vi "Objects bottom cords.vi"(2 "error in (no error)":errorcluster, 3 "Image":T4) -> (0 "error out":errorcluster, 1 "Objects bottom cords":T3(array[cluster]))   [LabVIEW 2009, in "ImageAnalysis.lvlib"]
doc: "Inputs:\nA binary image where white spotts are objects to detect.\n\nOutput:\nA 1-D array with a cluster element per detected object. Each cluster contains a 1-D array with the detected bottom points of the object."
uses:
  ImageAnalysis.lvlib
  <vilib>/vision/Image Controls.llb/IMAQ Image.ctl
  <vilib>/Analysis/Matrix/Numeric/Conversions/Array To Matrix - RA2.vi
  <vilib>/vision/NI_Vision_Development_Module.lvlib
  <vilib>/Analysis/Matrix/NI_Matrix.lvlib
panel:
  in  "Object":T1
  out "Rectangle":T2 {"Rotation" format="%.2f"; "Left" scale=0.0..1024.0; "Right" scale=0.0..1024.0; "Bottom" scale=1024.0..0.0; "Top" scale=1024.0..0.0}
  in  "Rectangle cluster":T2 {"Rotation" min=-90.0 max=90.0 step=1.0 format="%.2f"; "Left" scale=0.0..1024.0; "Right" scale=0.0..1024.0; "Bottom" scale=1024.0..0.0; "Top" scale=1024.0..0.0}
  # "Excecution time for this node is approx: 350 ms"
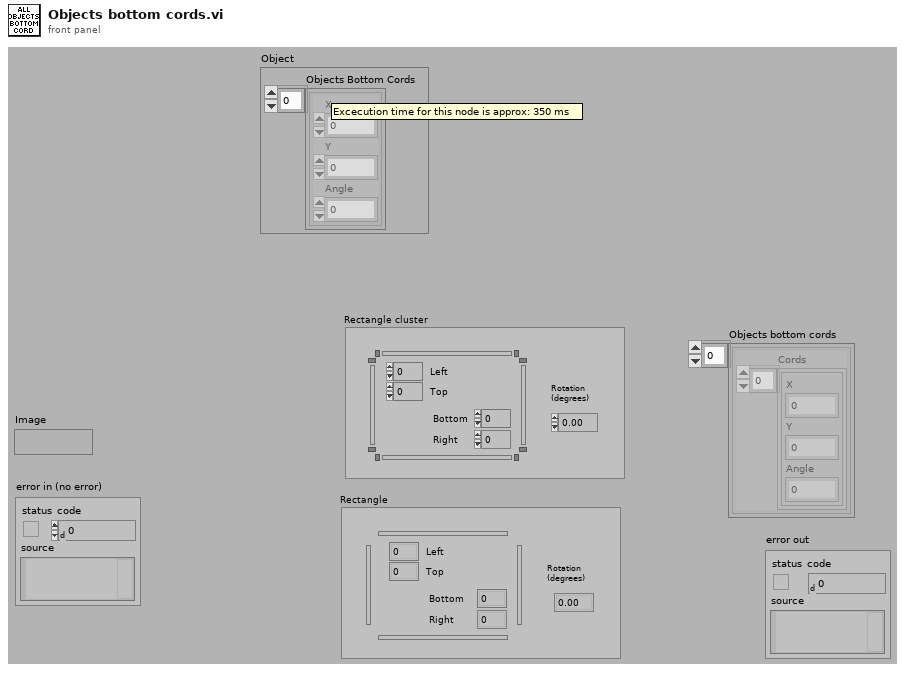
[diagram p1: front panel]
types:
  T1 = cluster{"Objects Bottom Cords":cluster{"X":dbl, "Y":dbl, "Angle":dbl}[]}
  T2 = typedef "IMAQ Rectangle" = cluster{"Left":i32, "Top":i32, "Right":i32, "Bottom":i32, "Rotation":dbl}
  T3 = cluster{"Cords":cluster{"X":dbl, "Y":dbl, "Angle":dbl}[]}[]
  T4 = typedef "IMAQ Image.ctl" = refnum<image>
  T5 = typedef "Particle Parameters" = i32
  T6 = typedef "Image Type" = u32
  T7 = cluster{"Objects Bottom Cords":cluster{"X":dbl, "Y":dbl, "Angle":dbl}[]}[]
  T8 = typedef "NI_Matrix.lvlib/RealMatrix.ctl" = dbl[][]
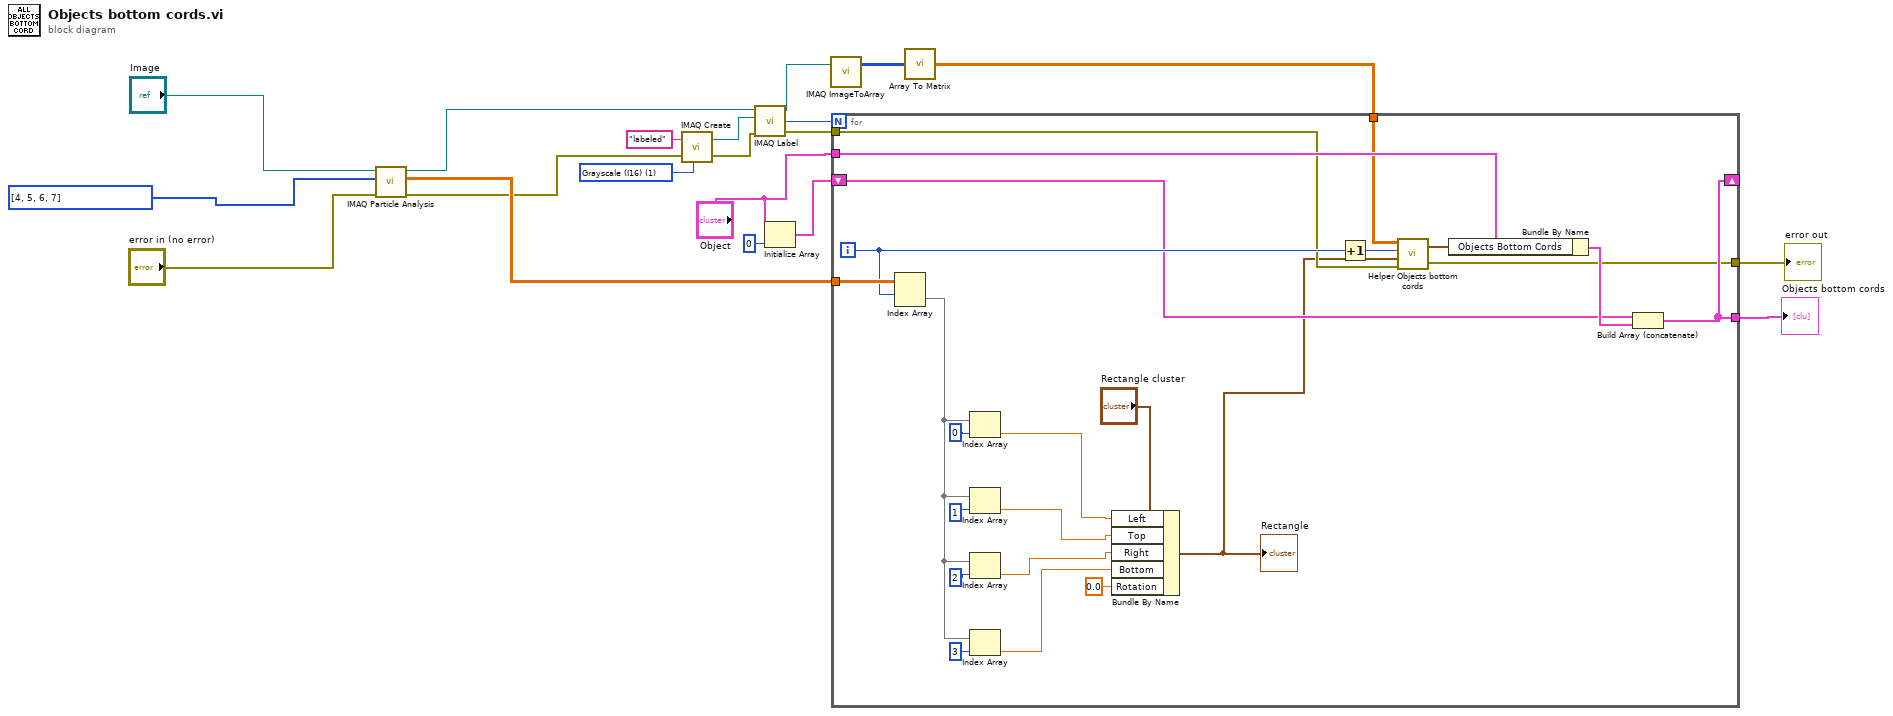
[diagram p0: block diagram]
diagram:
  w5 = T5[] [4, 5, 6, 7] items=["Center of Mass X", "Center of Mass Y", "First Pixel X", "First Pixel Y", "Bounding Rect Left", "Bounding Rect Top", "Bounding Rect Right", "Bounding Rect Bottom", "Max Feret Diameter Start X", "Max Feret Diameter Start Y", "Max Feret Diameter End X", "Max Feret Diameter End Y", "Max Horiz. Segment Length Left", "Max Horiz. Segment Length Right", "Max Horiz. Segment Length Row", "-", "Bounding Rect Width", "Bounding Rect Height", "Bounding Rect Diagonal", "Perimeter", "Convex Hull Perimeter", "Holes' Perimeter", "Max Feret Diameter", "Equivalent Ellipse Major Axis", "Equivalent Ellipse Minor Axis", "Equivalent Ellipse Minor Axis (Feret)", "Equivalent Rect Long Side", "Equivalent Rect Short Side", "Equivalent Rect Diagonal", "Equivalent Rect Short Side (Feret)", "Average Horiz. Segment Length", "Average Vert. Segment Length", "Hydraulic Radius", "Waddel Disk Diameter", "-", "Area", "Holes' Area", "Particle & Holes' Area", "Convex Hull Area", "Image Area", "-", "Number of Holes", "Number of Horiz. Segments", "Number of Vert. Segments", "-", "Orientation", "Max Feret Diameter Orientation", "-", "% Area/Image Area", "% Area/(Particle & Holes' Area)", "Ratio of Equivalent Ellipse Axes", "Ratio of Equivalent Rect Sides", "-", "Elongation Factor", "Compactness Factor", "Heywood Circularity Factor", "Type Factor", "-", "Sum X", "Sum Y", "Sum XX", "Sum XY", "Sum YY", "Sum XXX", "Sum XXY", "Sum XYY", "Sum YYY", "-", "Moment of Inertia XX", "Moment of Inertia XY", "Moment of Inertia YY", "Moment of Inertia XXX", "Moment of Inertia XXY", "Moment of Inertia XYY", "Moment of Inertia YYY", "Norm. Moment of Inertia XX", "Norm. Moment of Inertia XY", "Norm. Moment of Inertia YY", "Norm. Moment of Inertia XXX", "Norm. Moment of Inertia XXY", "Norm. Moment of Inertia XYY", "Norm. Moment of Inertia YYY", "Hu Moment 1", "Hu Moment 2", "Hu Moment 3", "Hu Moment 4", "Hu Moment 5", "Hu Moment 6", "Hu Moment 7"] ("Pixel Measurements")
  w16 = T6 1 items=["Grayscale (U8)", "Grayscale (I16)", "Grayscale (SGL)", "Complex (CSG)", "RGB (U32)", "HSL (U32)", "RGB (U64)", "Grayscale (U16)"] ("Image Type")
  n1 = call "IMAQ Particle Analysis"("error in (no error)"="error in (no error)", "Pixel Measurements"=w5, "Image"="Image") -> ("error out"=w4:errorcluster, "Particle Measurements (Pixels)"=w10:dbl[][], "Image Out (duplicate)"=w18:T4)  [unwired: 3 in, 3 out]
  n2 = call "IMAQ Create"("Image Name"="labeled", "Image Type"=w16, "error in (no error)"=w4) -> ("New Image"=w15:T4, "error out"=w3:errorcluster)  [unwired: 2 in]
  n3 = call "IMAQ Label"("error in (no error)"=w3, "Image Dst"=w15, "Image Src"=w18) -> ("error out"=w2:errorcluster, "Number of Particles"=w12:i32, "Image Dst Out"=w14:T4)  [unwired: 1 in]
  n4 = Initialize Array("Object", 0 ("dimension size")) -> (w7:T7)
  n5 = call "IMAQ ImageToArray"("Image"=w14) -> ("Image Pixels (I16)"=w13:i16[][])  [unwired: 3 in, 4 out]
  n6 = call-poly <vilib>:"Array To Matrix.vi"("Real 2D Array"=w13) -> ("Real Matrix"=w9:T8)
  n7 = for {
    N: w12 -> [_]
    tunnel: [w27] -> w11
    tunnel: w10 -> [w30]
    tunnel: w9 -> [w23]
    shift-right: [w27] -> _
    shift-left: w7 -> [w28]
    tunnel: "Object" -> [w26]
    tunnel: w2 -> [w25]
    tunnel: [w24] -> w1
    i -> [w29]
    n8 = Index Array(array=w30, index (row)=w29) -> (element=w31:dbl[])  [unwired: 1 in]
    n9 = Index Array(array=w31, index=0) -> (element=w32:dbl)
    n10 = Index Array(array=w31, index=1) -> (element=w33:dbl)
    n11 = Index Array(array=w31, index=2) -> (element=w34:dbl)
    n12 = Index Array(array=w31, index=3) -> (element=w35:dbl)
    n13 = Bundle By Name(cluster="Rectangle cluster", "Left"=w32, "Top"=w33, "Right"=w34, "Bottom"=w35, "Rotation"=0.0) -> (w22:T2)
    "Rectangle" <- w22
    n14 = Increment(x=w29) -> (x+1=w43:i32)
    n15 = call "Helper Objects bottom cords.vi"("error in (no error)"=w25, "Rectangle"=w22, "Object color"=w43, "Image matrix"=w23) -> ("error out"=w24:errorcluster, "Objects Bottom Cords"=w21:cluster{"X":dbl, "Y":dbl, "Angle":dbl}[])
    n16 = Bundle By Name(cluster=w26, "Objects Bottom Cords"=w21) -> (w42:T1)
    n17 = Build Array (concatenate)(w28, w42) -> (w27:T7)
  }
  "Objects bottom cords" <- w11
  "error out" <- w1
